vi "Chart-Single.vi"() -> ()   [LabVIEW 2020]
panel:
  in  "Delay":u32=100
  out "Chart-Strip":dbl(graph)
  out "Chart-Sweep":dbl(graph)
  out "Chart-Scope":dbl(graph)
  in  "Stop":bool
  # "ms"
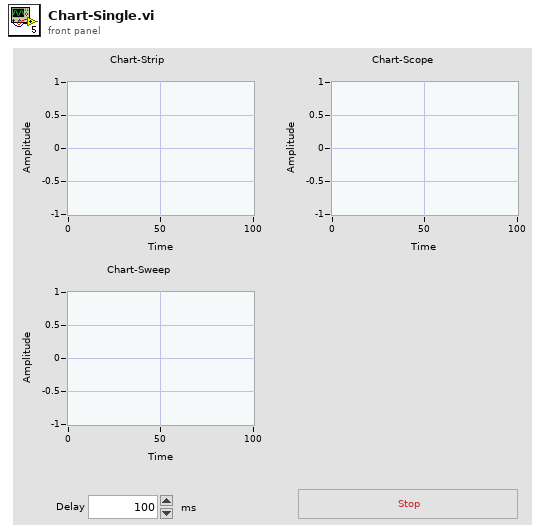
[diagram p1: front panel]
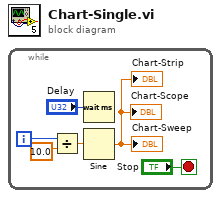
[diagram p0: block diagram]
diagram:
  n1 = while {
    i -> [w5]
    stop <- "Stop" stop-if-true
    n2 = Divide(x=w5, y=10.0 ("x")) -> (x/y=w3:dbl)
    n3 = Wait (ms)(milliseconds to wait="Delay") -> ()  [unwired: 1 out]
    n4 = Sine(x=w3) -> (sin(x)=→"Chart-Scope" →"Chart-Sweep" →"Chart-Strip":dbl)
  }
